vi "I64ToString(cast).vi"(1 "I64":i64 format="DEC:%2d\nHEX:%2x") -> (0 "String":string)   [LabVIEW 2012]
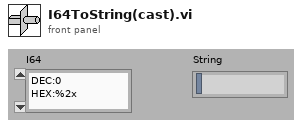
[diagram p1: front panel]
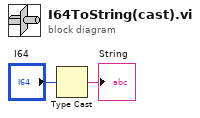
[diagram p0: block diagram]
diagram:
  n1 = Type Cast(x="I64") -> (*(type *) &x=→"String":string)  [unwired: 1 in]
